vi "FromIScan.vi"(10 "OfficeTron3000.lvlib:OT3IScan.lvclass":refnum<class "OT3IScan.lvclass">) -> (3 "OfficeTron3000.lvlib:OfficeTron3000.lvclass":refnum<class "OfficeTron3000.lvclass">)   [LabVIEW 2018, in "OfficeTron3000.lvlib" / "OfficeTron3000.lvclass"]
uses:
  OfficeTron3000.lvclass
  OT3IScan/OT3IScan.lvclass
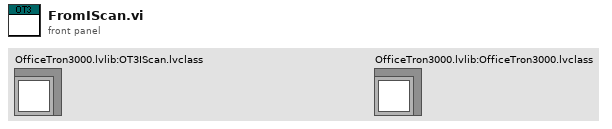
[diagram p1: front panel]
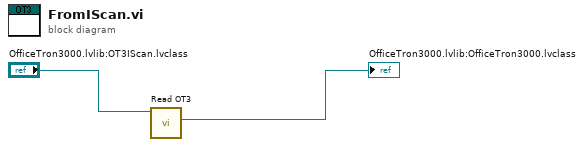
[diagram p0: block diagram]
diagram:
  n1 = call "Read OT3.vi"("OT3IScan in"="OfficeTron3000.lvlib:OT3IScan.lvclass") -> ("OT3"=→"OfficeTron3000.lvlib:OfficeTron3000.lvclass":refnum<class "OfficeTron3000.lvclass">)  [unwired: 9 in, 1 out]
